vi "Swerve Wheel.vi"(2 "Wheel":T1(ring), 3 "Debug?":bool, 4 "Inputs":dbl[](array[numeric])) -> (0 "Speed":dbl)   [LabVIEW 2016, in "CAN Talon SRX Swerve.lvlib"]
uses:
  CAN Talon SRX Swerve.lvlib
  <vilib>/Rock Robotics/WPI/ThirdParty/CanMotor/TalonSRX/WPI_CANTalonSRX_APIControlMode.ctl
  <vilib>/Rock Robotics/Network Tables/NT Read Number.vi
  <vilib>/addons/control/pid/pid.llb/PID (DBL).vi
  <vilib>/addons/control/pid/NI_PID_pid.lvlib
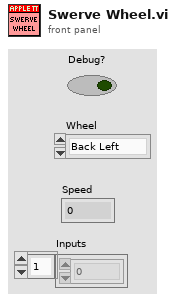
[diagram p1: front panel]
types:
  T1 = enum16{"Back Left", "Back Right", "Front Left", "Front Right"}
  T2 = typedef "WPI_CANTalonSRX_APIControlMode.ctl" = enum8{"Percent VBus", "Speed", "Position", "Slave", "Unchanged / Invalid", "Voltage Compensation", "Current", "Motion Profile", "Motion Magic"}
  T3 = enum16{"Z", "Y", "X", "Rot. Point X", "Rot. Point Y", "Width/2", "Max", "Length/2"}
  T4 = enum16{"Z Axis", "Y", "X", "Rot. Point X", "Rot. Point Y", "Width/2", "Max", "Length/2"}
  T5 = cluster{"proportional gain (Kc)":dbl, "integral time (Ti, min)":dbl, "derivative time (Td, min)":dbl}
  T6 = typedef "WPI_AnalogChannelDevRef.ctl" = cluster{"DevStatus":errorcluster, "Analog Channel":T7}
  T7 = typedef "FPGA_AIChannel.ctl" = enum8{"AI 0", "AI 1", "AI 2", "AI 3", "AI MXP 0", "AI MXP 1", "AI MXP 2", "AI MXP 3", "Invalid"}
  T8 = typedef "WPI_MotorControlDeviceRef.ctl" = cluster{"DeviceStatus":errorcluster, "Type":T9, "PWM":cluster{"PWM Channel":T10, "DeadBand":T11}, "CAN":cluster{"Device Number":u8, "SetOutput VI Ref":variant, "GetOutput VI Ref":variant, "Enable VI Ref":variant, "Disable VI Ref":variant, "Data":variant}, "Invert":bool}
  T9 = typedef "WPI_MotorControlType.ctl" = enum16{"PWM", "CAN"}
  T10 = typedef "FPGA_DIOPWMChannel.ctl" = enum8{"PWM 0", "PWM 1", "PWM 2", "PWM 3", "PWM 4", "PWM 5", "PWM 6", "PWM 7", "PWM 8", "PWM 9", "PWM MXP 0", "PWM MXP 1", "PWM MXP 2", "PWM MXP 3", "PWM MXP 4", "PWM MXP 5", "PWM MXP 6", "PWM MXP 7", "PWM MXP 8", "PWM MXP 9", "Invalid"}
  T11 = typedef "WPI_PWMDeadband.ctl" = cluster{"Name":string, "maxPositivePwm":i32, "minPositivePwm":i32, "centerPwm":i32, "maxNegativePwm":i32, "minNegativePwm":i32, "angularRange":u16}
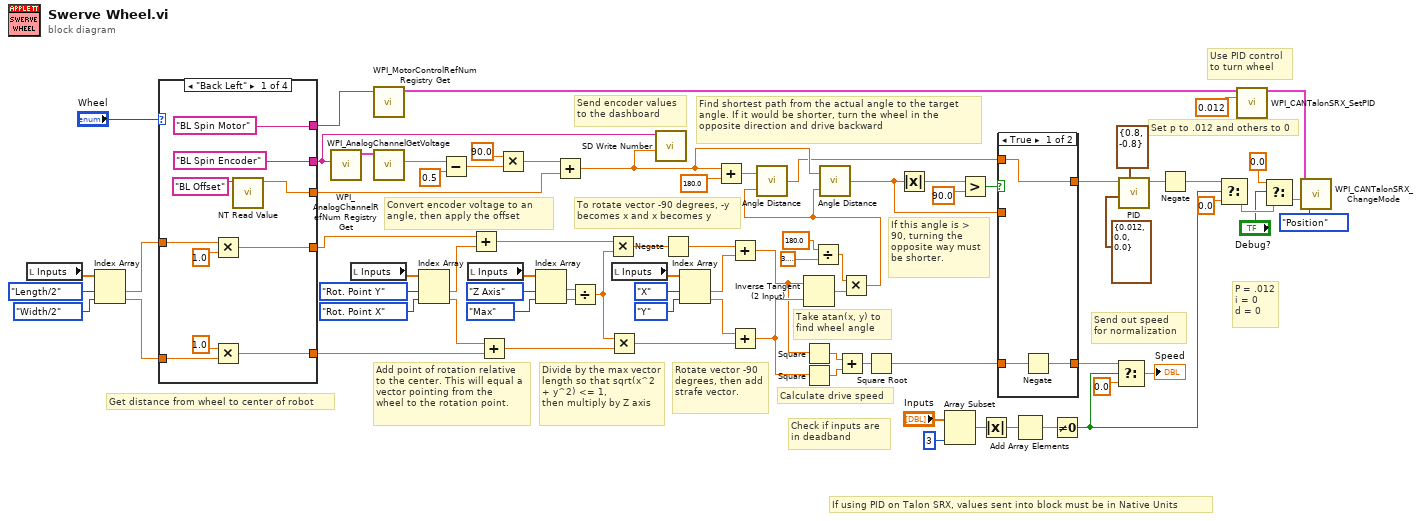
[diagram p0: block diagram]
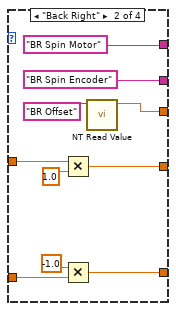
[diagram p3: hidden frame]
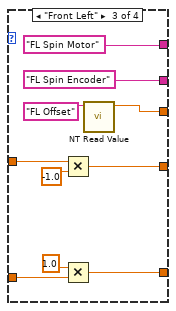
[diagram p4: hidden frame]
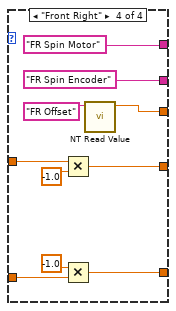
[diagram p5: hidden frame]
diagram:
  # "If using PID on Talon SRX, values sent into block must be in Native Units"
  # "Set p to .012 and others to 0"
  # "P = .012\ni = 0\nd = 0"
  # "Send encoder values \nto the dashboard"
  # "To rotate vector -90 degrees, -y becomes x and x becomes y"
  # "Divide by the max vector length so that sqrt(x^2 + y^2) <= 1,\nthen multiply by Z axis"
  # "Add point of rotation relative to the center. This will equal a vector pointing from the\nwheel to the rotation point."
  # "Send out speed\nfor normalization"
  # "Check if inputs are\nin deadband"
  # "Convert encoder voltage to an angle, then apply the offset"
  # "If this angle is > 90, turning the opposite way must be shorter."
  # "Use PID control\nto turn wheel"
  # "Find shortest path from the actual angle to the target angle. If it would be shorter, turn the wheel in the opposite direction and drive backward"
  # "Take atan(x, y) to find wheel angle"
  # "Calculate drive speed"
  # "Rotate vector -90 degrees, then add strafe vector."
  # "Get distance from wheel to center of robot"
  n1 = local read "Inputs"() -> (w19:dbl[])
  n2 = Index Array(array=w19, index #1=T3."Length/2", index #2=T3."Width/2") -> (element #1=w17:dbl, element #2=w16:dbl)
  n3 = case shown="\"Back Left\"" "Wheel" {
    tunnel: ["BL Spin Encoder" "BR Spin Encoder" "FL Spin Encoder" "FR Spin Encoder"] -> w46
    tunnel: ["BL Spin Motor" "BR Spin Motor" "FL Spin Motor" "FR Spin Motor"] -> w66
    tunnel: [w87 w97 w107 w117] -> w56
    tunnel: w17 -> [w85 w95 w105 w115]
    tunnel: w16 -> [w83 w93 w103 w113]
    tunnel: [w82 w92 w102 w112] -> w43
    tunnel: [w81 w91 w101 w111] -> w39
    frame "Back Left" {
      n4 = Multiply(x=w85, y=1.0) -> (x*y=w82:dbl)
      n5 = Multiply(x=1.0 ("y"), y=w83) -> (x*y=w81:dbl)
      n6 = call-poly <vilib>:"NT Read Value.vi"("Name"="BL Offset") -> ("Numeric"=w87:dbl)  [unwired: 9 in, 1 out]
    }
    frame "Back Right" {
      n7 = Multiply(x=w95, y=1.0) -> (x*y=w92:dbl)
      n8 = Multiply(x=-1.0 ("y"), y=w93) -> (x*y=w91:dbl)
      n9 = call-poly <vilib>:"NT Read Value.vi"("Name"="BR Offset") -> ("Numeric"=w97:dbl)  [unwired: 9 in, 1 out]
    }
    frame "Front Left" {
      n10 = Multiply(x=w105, y=-1.0) -> (x*y=w102:dbl)
      n11 = Multiply(x=1.0 ("y"), y=w103) -> (x*y=w101:dbl)
      n12 = call-poly <vilib>:"NT Read Value.vi"("Name"="FL Offset") -> ("Numeric"=w107:dbl)  [unwired: 9 in, 1 out]
    }
    frame "Front Right" {
      n13 = Multiply(x=w115, y=-1.0) -> (x*y=w112:dbl)
      n14 = Multiply(x=-1.0 ("y"), y=w113) -> (x*y=w111:dbl)
      n15 = call-poly <vilib>:"NT Read Value.vi"("Name"="FR Offset") -> ("Numeric"=w117:dbl)  [unwired: 9 in, 1 out]
    }
  }
  n16 = call <vilib>:"WPI_AnalogChannelRefNum Registry Get.vi"("refnum name"=w46) -> ("AIDeviceRef"=w61:T6)  [unwired: 9 in, 1 out]
  n17 = local read "Inputs"() -> (w41:dbl[])
  n18 = call <vilib>:"WPI_MotorControlRefNum Registry Get.vi"("refnum name"=w66) -> ("MotorControlDevRef"=w4:T8)  [unwired: 9 in, 1 out]
  n19 = call <vilib>:"WPI_AnalogChannelGetVoltage.vi"("AIDeviceRef"=w61) -> ("Voltage"=w60:dbl)  [unwired: 8 in, 2 out]
  n20 = Index Array(array=w41, index #1=T3."Rot. Point Y", index #2=T3."Rot. Point X") -> (element #1=w37:dbl, element #2=w38:dbl)
  n21 = Subtract(x=w60, y=0.5) -> (x-y=w59:dbl)
  n22 = local read "Inputs"() -> (w35:dbl[])
  n23 = Add(x=w43, y=w37) -> (x+y=w12:dbl)
  n24 = Add(x=w38, y=w39) -> (x+y=w31:dbl)
  n25 = Multiply(x=90.0 ("y"), y=w59) -> (x*y=w57:dbl)
  n26 = Index Array(array=w35, index #1=T4."Z Axis", index #2=T3."Max") -> (element #1=w32:dbl, element #2=w33:dbl)
  n27 = Add(x=w57, y=w56) -> (x+y=w10:dbl)
  n28 = Divide(x=w32, y=w33) -> (x/y=w30:dbl)
  n29 = Multiply(x=w12, y=w30) -> (x*y=w14:dbl)
  n30 = Multiply(x=w30, y=w31) -> (x*y=w25:dbl)
  n31 = local read "Inputs"() -> (w28:dbl[])
  n32 = call <vilib>:"SD Write Number.vi"("Numeric"=w10, "Name"=w46) -> ()  [unwired: 8 in, 2 out]
  n33 = Negate(x=w14) -> (-x=w13:dbl)
  n34 = Index Array(array=w28, index #1=T3."X", index #2=T3."Y") -> (element #1=w23:dbl, element #2=w24:dbl)
  n35 = Add(x=w10, y=180.0 ("f")) -> (x+y=w53:dbl)
  n36 = Add(x=w13, y=w23) -> (x+y=w21:dbl)
  n37 = Add(x=w24, y=w25) -> (x+y=w22:dbl)
  n38 = Inverse Tangent (2 Input)(1:w22, 2:w21) -> (0:w77:dbl)
  n39 = Square(x=w21) -> (x^2=w26:dbl)
  n40 = Square(x=w22) -> (x^2=w76:dbl)
  n41 = Divide(x=180.0 ("y"), y=3.141592653589793) -> (x/y=w74:dbl)
  n42 = Add(x=w26, y=w76) -> (x+y=w75:dbl)
  n43 = Multiply(x=w74, y=w77) -> (x*y=w15:dbl)
  n44 = call "Angle Distance.vi"("target angle"=w15, "current angle"=w53) -> ("distance"=w9:dbl)
  n45 = call "Angle Distance.vi"("target angle"=w15, "current angle"=w10) -> ("distance"=w68:dbl)
  n46 = Square Root(x=w75) -> (sqrt(x)=w67:dbl)
  n47 = Absolute Value(x=w68) -> (abs(x)=w69:dbl)
  n48 = Array Subset(array="Inputs", length=3) -> (w52:dbl[])  [unwired: 1 in]
  n49 = Greater?(x=w69, y=90.0) -> (0:w48:bool)
  n50 = Absolute Value(x=w52) -> (abs(x)=w44:dbl[])
  n51 = case shown="True" w48 {
    tunnel: w9 -> [w121 _]
    tunnel: w68 -> [_ w125]
    tunnel: [w122 w124] -> w51
    tunnel: w67 -> [w123 w124]
    tunnel: [w121 w125] -> w63
    frame True {
      n52 = Negate(x=w123) -> (-x=w122:dbl)
    }
    frame False {
    }
  }
  n53 = Add Array Elements(numeric array=w44) -> (sum=w78:dbl)
  n54 = Not Equal To 0?(x=w78) -> (x != 0?=w47:bool)
  n55 = Select(t=w51, s=w47, f=0.0) -> (s? t:f=→"Speed":dbl)
  n56 = call-poly <vilib>:"PID.vi"("output range"=cluster{"output high":dbl, "output low":dbl} {"output high"=0.8, "output low"=-0.8}, "PID gains"=T5 {"proportional gain (Kc)"=0.012, "integral time (Ti, min)"=0.0, "derivative time (Td, min)"=0.0}, "setpoint"=w63) -> ("output"=w55:dbl)  [unwired: 7 in, 1 out]
  n57 = Negate(x=w55) -> (-x=w45:dbl)
  n58 = Select(t=w45, s=w47, f=0.0) -> (s? t:f=w7:dbl)
  n59 = call <vilib>:"WPI_CANTalonSRX_SetPID.vi"("CAN Talon SRX Ref"=w4, "P"=0.012) -> ("CAN Talon SRX Ref"=w3:T8)  [unwired: 12 in, 1 out]
  n60 = Select(t=0.0, s="Debug?", f=w7) -> (s? t:f=w6:dbl)
  n61 = call <vilib>:"WPI_CANTalonSRX_ChangeMode.vi"("Output"=w6, "Control Mode"=WPI_CANTalonSRX_APIControlMode."Position", "CAN Talon SRX Ref"=w3) -> ()  [unwired: 7 in, 2 out]
